vi "viewport.vi"(4 "Error In":errorcluster={"status"=FALSE, "code"=0, "source"="\"weather configured to \\\"Default\\\"\","}, 7 "Viewport Camera configuration":string="{\n  \"type\": \"ViewportCamera\",\n  \"listen_port\": 0,\n  \"server_ip\": \"127.0.0.1\",\n  \"server_port\":8999,\n  \"description\": \"\",\n  \"location\": {\n      \"x\":  -400.0,\n      \"y\": 0.0,\n      \"z\": 300.0\n    },\n    \"rotation\": {\n      \"pitch\": -15.0,\n      \"yaw\": 0.0,\n      \"roll\": 0.0\n    },\n    \"stream_dimensions\": {\n      \"x\": 512.0,\n      \"y\": 512.0\n    },\n   \"enable_streaming\": false,\n   \"use_vehicle_hud\": false,\n   \"wait_for_fresh_frame\": true,\n   \"sensor_size\": 9.069999694824219,\n    \"dynamic_range\": 50,\n    \"fov\": 60.0,\n    \"focal_length\": 9.0,\n    \"fstop\": 1.4,\n    \"max_distance\": 50000.0,\n    \"min_shutter\": 0.000500,\n    \"max_shutter\": 0.001400,\n    \"sensor_size\": 9.07,\n    \"channels\": \"bgra\",\n    \"channel_depth\": 1,\n    \"annotation\": {\n        \"cull_partial_frame\": false,\n        \"debug_draw\": false,\n        \"desired_tags\": [],\n        \"far_plane\": 10000.0,\n        \"include_annotation\": false,\n        \"include_obb\": false,\n        \"include_tags\": false\n    }\n}") -> (0 "Error Out":errorcluster={"status"=FALSE, "code"=0, "source"="\"complete\","})   [LabVIEW 2019]
doc: "Configures the camera on the Viewport"
uses:
  tools/simx_common.vi
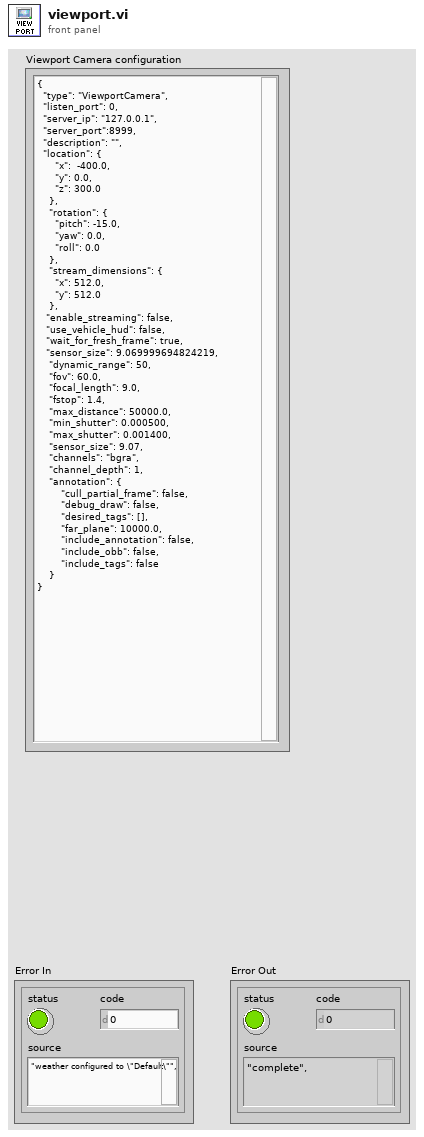
[diagram p1: front panel]
types:
  T1 = typedef "simx_connection.ctl" = cluster{"Config":T2, "Connections":T5, "Map":cluster{"lanes":cluster{"x":dbl[], "y":dbl[], "z":dbl[]}, "StartPosition":cluster{"start_points":T6, "StartRotation":dbl[], "StartLocation":dbl[]}, "Draw Map Size":T7, "DrawArea":cluster{"min_Y":dbl, "min_X":dbl, "Scale X":dbl, "Scale Y":dbl}, "Map":picture, "Map Geojson":string}}
  T2 = typedef "config.ctl" = cluster{"Trajectory":T3, "Weather":T4}
  T3 = typedef "trajectory.ctl" = cluster{"Number of frames":i32, "Frame number":i32, "Trajectory":string}
  T4 = typedef "weather.ctl" = cluster{"id":string}
  T5 = typedef "connections.ctl" = cluster{"Simulator Connection":refnum<k5>, "server_ip":string, "Port":i32, "Sensor connections":refnum<k5>[]}
  T6 = typedef "start_points.ctl" = cluster{"locations":dbl[][], "rotations":dbl[][], "type":string[]}
  T7 = typedef "LVBoundsTypeDef.ctl" = cluster{"Width":u32, "Height":u32}
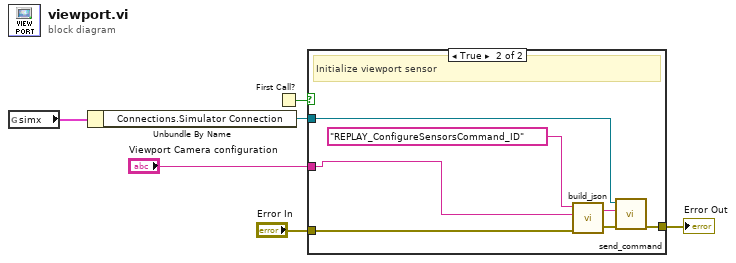
[diagram p0: block diagram]
diagram:
  n1 = global read "simx_common.vi" "simx"() -> (w1:T1)
  n2 = Unbundle By Name(w1) -> ("Connections.Simulator Connection"=w5:refnum<k5>)
  n3 = First Call?() -> (First Call?: T/F=w2:bool)
  n4 = case shown="True" w2 {
    tunnel: [w7 w9] -> w4
    tunnel: "Viewport Camera configuration" -> [_ w8]
    tunnel: "Error In" -> [w7 w10]
    tunnel: w5 -> [_ w11]
    frame False {
      # "Nothing to sample"
    }
    frame True {
      # "Initialize viewport sensor"
      n5 = call "build_json.vi"("error in"=w10, "Message"=w8, "Command_ID"="REPLAY_ConfigureSensorsCommand_ID") -> ("error out"=w12:errorcluster, "JSON Out"=w13:string)  [unwired: 1 in]
      n6 = call "send_command.vi"("error in"=w12, "JSON Command"=w13, "TCP Network Connection in"=w11) -> ("error out"=w9:errorcluster)  [unwired: 1 in, 3 out]
    }
  }
  "Error Out" <- w4
